vi "GetRectIntersection.vi"(8 "No Error":errorcluster, 10 "B":T1, 11 "A":T1) -> (0 "Error Out":errorcluster, 2 "Intersection":T1, 3 "Intersect?":bool)   [LabVIEW 2026, in "SDL3.lvlib" / "Rect.lvlib"]
doc: "<B>Summary</B>\nCalculate the intersection of two rectangles."
uses:
  Rect.lvlib
  Rect--cluster.ctl
  Lib/SDL3.dll
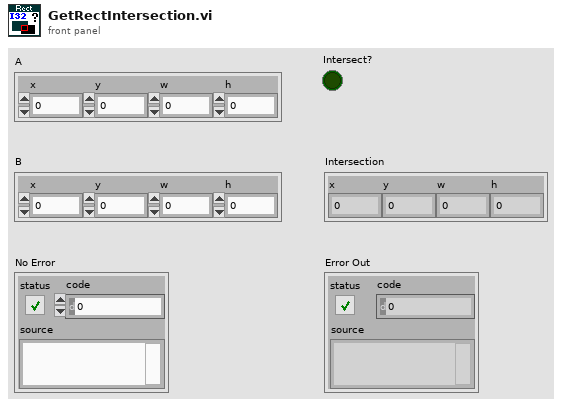
[diagram p1: front panel]
types:
  T1 = typedef "SDL3.lvlib/Rect.lvlib/Rect--cluster.ctl" = cluster{"x":i32, "y":i32, "w":i32, "h":i32}
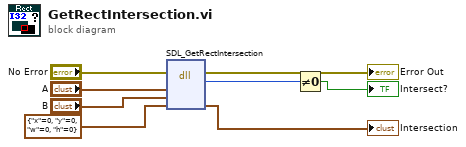
[diagram p0: block diagram]
diagram:
  n1 = dll-call lib="C:/Users/saukko/Dev/LV-SDL3/Sources/SDL3/Lib/SDL3.*" fn="SDL_GetRectIntersection"(error in="No Error", "A"="A", "B"="B", "result"=T1 {"x"=0, "y"=0, "w"=0, "h"=0} ("B")) -> (error out=→"Error Out":errorcluster, "return type"=w6:i32, "result"=→"Intersection":T1)  [unwired: 4 in, 1 out]
  n2 = Not Equal To 0?(x=w6) -> (x != 0?=→"Intersect?":bool)
